vi "Load Virt Instrs.vi"(7 "Target Enqueuer":refnum<class "Message Enqueuer.lvclass">, 8 "error in":errorcluster, 10 "Virt Instrs":T1(array[cluster]), 11 "MSS in":refnum<class "Measure and Stimulus Subsystems.lvclass">) -> (0 "error out":errorcluster, 3 "MSS out":refnum<class "Measure and Stimulus Subsystems.lvclass">)   [LabVIEW 2023, in "HAL GOOP4.lvlib" / "Measure and Stimulus Subsystems.lvclass"]
uses:
  Measure and Stimulus Subsystems.lvclass
  <vilib>/ActorFramework/Message Enqueuer/Message Enqueuer.lvclass
  Measure and Stimulus Subsystems.lvclass/Measure and Stimulus Subsystems.ctl
  Virt Instr Host/Virt Instr Local.lvclass
  Virt Instr Base/Virt Instr Base.lvclass/Virt Instr Base.ctl
  <vilib>/Utility/miscctls.llb/LVMapReplaceAction.ctl
  Virt Instr Target/Virt Instr Target.lvclass
  MSS Target/IMSS Target Actor Messages/Init Virtual Instruments Msg/Init Virtual Instruments Msg.lvclass/Init Virtual Instruments Msg.ctl
  <vilib>/ActorFramework/Message Enqueuer/Message Enqueuer.lvclass/Message Enqueuer.ctl
  <vilib>/ActorFramework/Message Enqueuer/Enqueue.vi
  MSS Target/IMSS Target Actor Messages/Init Virtual Instruments Msg/Init Virtual Instruments Msg.lvclass
  <vilib>/Utility/LVClass/Get LV Class Name.vi
  <resource>/AFDebug/Generate Trace for Message.vi
  <vilib>/ActorFramework/Message Priority Queue/Priority Enqueue.vi
  Virt Instr Base/Virt Instr Base.lvclass
  D:/git/HAL/HAL GOOP4/Virt Instr Base/Virt Instr Base.lvclass
  D:/git/HAL/HAL GOOP4/Virt Instr Host/Virt Instr Local.lvclass
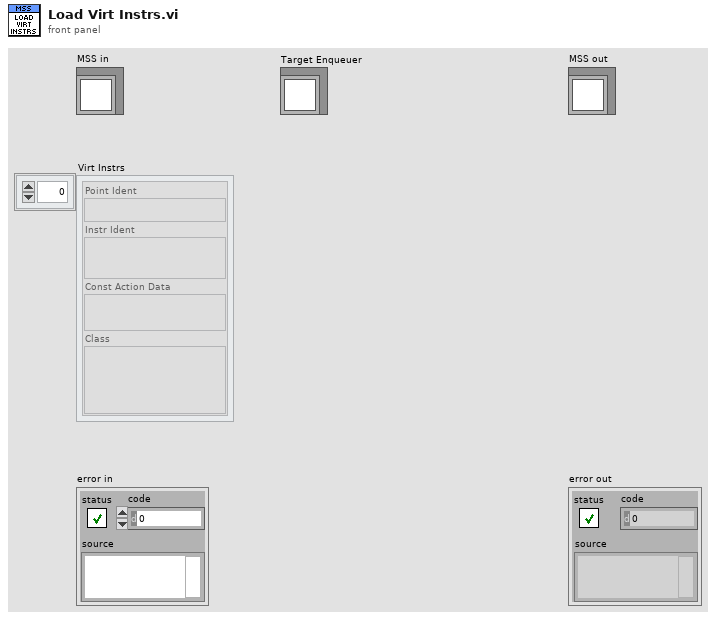
[diagram p1: front panel]
types:
  T1 = cluster{"Point Ident":string, "Instr Ident":string, "Const Action Data":string, "Class":string}[]
  T2 = typedef "LVMapReplaceAction.ctl" = enum32{"Modify Entry only if found", "Add or Modify Entry", "Delete Entry"}
  T3 = map{string, refnum<class "Virt Instr Local.lvclass">}
  T4 = map{string, cluster{"Instrument":refnum<class "Instrument.lvclass">, "Ref Count":u8}}
  T5 = cluster{"Instrument":refnum<class "Instrument.lvclass">, "Ref Count":u8}
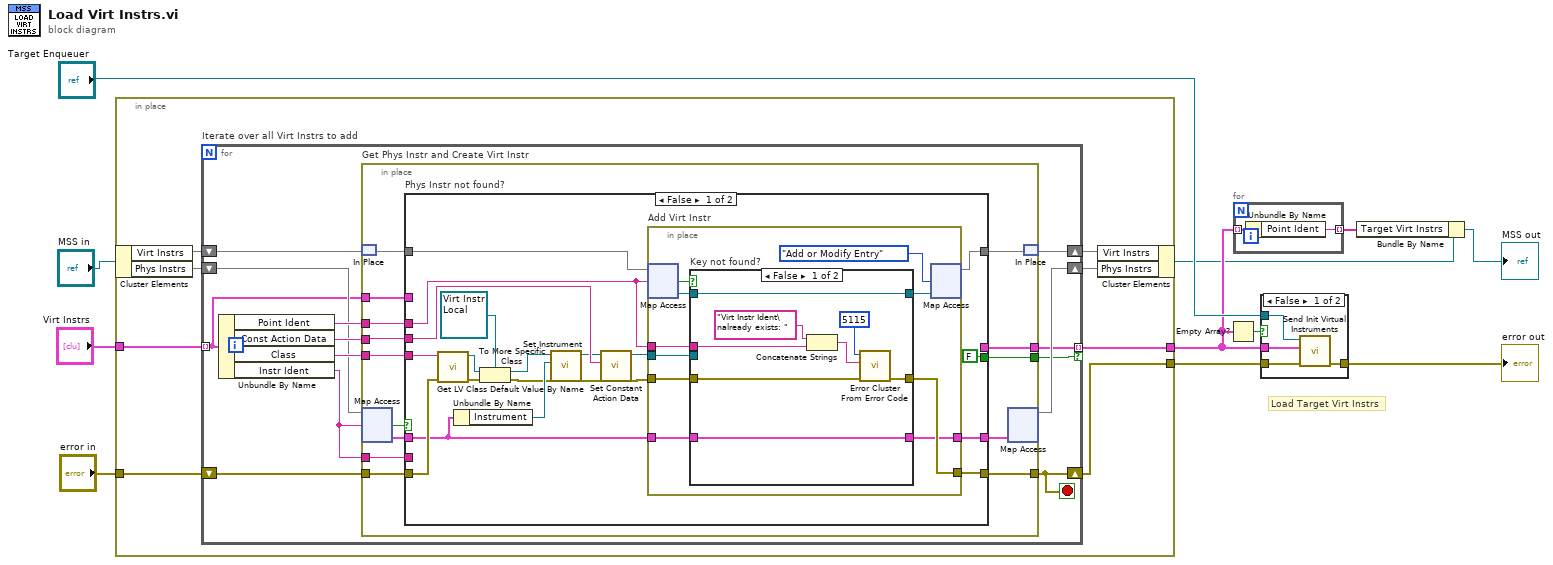
[diagram p0: block diagram]
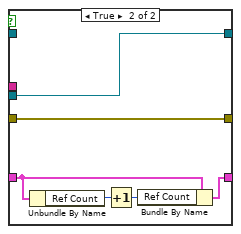
[diagram p2: hidden frame]
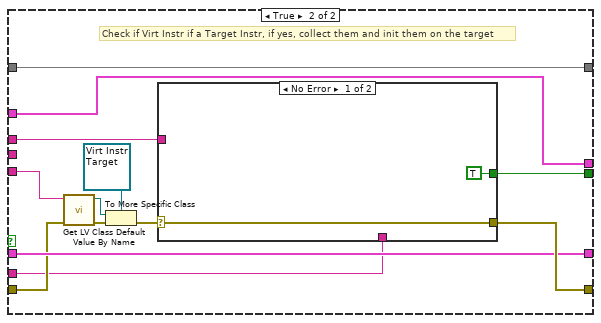
[diagram p3: hidden frame]
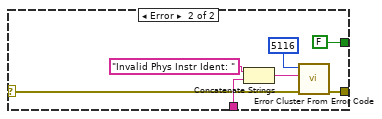
[diagram p4: hidden frame]
diagram:
  # "Load Target Virt Instrs"
  n1 = in-place {
    in-place-border: "error in" -> [w14]
    in-place-border: "Virt Instrs" -> [w19]
    in-place-border: [w13] -> w4
    in-place-border: [w12] -> w6
    n2 = in-place-cluster #1("MSS in") -> ("Virt Instrs"=w17:T3, "Phys Instrs"=w18:T4)
    n3 = for "Iterate over all Virt Instrs to add" {
      tunnel: w19 -> [w23] mode=indexing
      shift-right: [w29] -> w12
      shift-left: w14 -> [w31]
      shift-right: [w24] -> w15
      shift-left: w18 -> [w27]
      shift-right: [w25] -> w16
      shift-left: w17 -> [w26]
      tunnel: [w22] -> w13 mode=indexing if=w21
      stop <- w29 stop-if-true
      n4 = Unbundle By Name(w23) -> ("Point Ident"=w28:string, "Const Action Data"=w30:string, "Class"=w32:string, "Instr Ident"=w20:string)
      n5 = in-place "Get Phys Instr and Create Virt Instr" {
        in-place-border: w32 -> [w46]
        in-place-border: w31 -> [w45]
        in-place-border: w30 -> [w44]
        in-place-border: [w43] -> w29
        in-place-border: w28 -> [w42]
        in-place-border: w23 -> [w36]
        in-place-border: [w35] -> w22
        in-place-border: [w34] -> w21
        in-place-border: w20 -> [w33]
        n6 = in-place-match #2(w26) -> (w41:T3)
        n7 = in-place-map #3(w27, w20) -> (w39:T5, w37:bool)  [unwired: 1 in]
        n8 = case "Phys Instr not found?" shown="False" w37 {
          tunnel: w46 -> [w64 w97]
          tunnel: w45 -> [w63 w96]
          tunnel: w44 -> [w59 _]
          tunnel: [w56 w101] -> w43
          tunnel: w42 -> [w47 w91]
          tunnel: w41 -> [w53 w90]
          tunnel: [w58 w90] -> w40
          tunnel: w39 -> [w55 w100]
          tunnel: [w54 w100] -> w38
          tunnel: w36 -> [_ w93]
          tunnel: [_ w93] -> w35
          tunnel: [FALSE w92] -> w34
          tunnel: w33 -> [_ w89]
          frame False {
            n9 = call <vilib>:"Get LV Class Default Value By Name.vi"("error in (no error)"=w63, "class name"=w64) -> ("error out"=w62:errorcluster, "object"=w60:refnum<class>)  [unwired: 8 in]
            n10 = Unbundle By Name(w55) -> ("Instrument"=w51:refnum<class "Instrument.lvclass">)
            n11 = To More Specific Class(target class=refnum<class "Virt Instr Local.lvclass"> refnum ("Virt Instr Target"), reference=w60, error in=w62) -> (specific class reference=w50:refnum<class "Virt Instr Local.lvclass">, error out=w48:errorcluster)
            n12 = call "Set Instrument.vi"("HAL GOOP4.lvlib:Instrument"=w51, "Virt Instrument Base in"=w50) -> ("Virt Instrument Base out"=w52:refnum<class "Virt Instr Local.lvclass">)  [unwired: 9 in]
            n13 = call "Set Constant Action Data.vi"("Constant Action Data"=w59, "Virt Instr Base in"=w52) -> ("Virt Instr Base out"=w57:refnum<class "Virt Instr Local.lvclass">)  [unwired: 9 in]
            n14 = in-place "Add Virt Instr" {
              in-place-border: w57 -> [w72]
              in-place-border: w48 -> [w70]
              in-place-border: [w69] -> w56
              in-place-border: [w67] -> w54
              in-place-border: w55 -> [w66]
              in-place-border: w47 -> [w65]
              n15 = in-place-map #4(w53, w47) -> (w73:refnum<class "Virt Instr Local.lvclass">, w74:bool)  [unwired: 1 in]
              n16 = case "Key not found?" shown="False" w74 {
                tunnel: w73 -> [w81 _]
                tunnel: w72 -> [_ w83]
                tunnel: [w81 w83] -> w71
                tunnel: w70 -> [w82 w88]
                tunnel: [w79 w88] -> w69
                tunnel: w66 -> [w80 w85]
                tunnel: [w80 w84] -> w67
                tunnel: w65 -> [w75 _]
                frame False {
                  n17 = Concatenate Strings("Virt Instr Ident\nalready exists: " ("string"), w75) -> (w77:string)
                  n18 = call <vilib>:"Error Cluster From Error Code.vi"("error in (no error)"=w82, "error message (\"\")"=w77, "error code (0)"=5115) -> ("error out"=w79:errorcluster)  [unwired: 6 in]
                }
                frame True {
                  n19 = Unbundle By Name(w85) -> ("Ref Count"=w87:u8)
                  n20 = Increment(x=w87) -> (x+1=w86:u8)
                  n21 = Bundle By Name(cluster=w85, "Ref Count"=w86) -> (w84:T5)
                }
              }
              n22 = in-place-map #4(w71, LVMapReplaceAction."Add or Modify Entry" ("action")) -> (w58:T3)  [unwired: 2 out]
            }
          }
          frame True {
            # "Check if Virt Instr if a Target Instr, if yes, collect them and init them on the target"
            n23 = call <vilib>:"Get LV Class Default Value By Name.vi"("error in (no error)"=w96, "class name"=w97) -> ("error out"=w95:errorcluster, "object"=w99:refnum<class>)  [unwired: 8 in]
            n24 = To More Specific Class(target class=refnum<class "Virt Instr Target.lvclass"> refnum ("Virt Instr Target"), reference=w99, error in=w95) -> (error out=w94:errorcluster)  [unwired: 1 out]
            n25 = case shown="No Error" w94 {
              selector: w94 -> [w102 w104]
              tunnel: [w102 w110] -> w101
              tunnel: [TRUE FALSE] -> w92
              tunnel: w91 -> [_ _]
              tunnel: w89 -> [_ w106]
              frame No Error {
              }
              frame Error {
                n26 = Concatenate Strings("Invalid Phys Instr Ident: " ("string"), w106) -> (w105:string)
                n27 = call <vilib>:"Error Cluster From Error Code.vi"("error in (no error)"=w104, "error message (\"\")"=w105, "error code (0)"=5116) -> ("error out"=w110:errorcluster)  [unwired: 6 in]
              }
            }
          }
        }
        n28 = in-place-map #3(w38) -> (w24:T4)  [unwired: 1 in, 2 out]
        n29 = in-place-match #2(w40) -> (w25:T3)
      }
    }
    n30 = in-place-cluster #1("Virt Instrs"=w16, "Phys Instrs"=w15) -> (w3:refnum<class "Measure and Stimulus Subsystems.lvclass">)
  }
  n31 = Empty Array?(array=w4) -> (empty?=w8:bool)
  n32 = for {
    tunnel: [w112] -> w1 mode=indexing
    tunnel: w4 -> [w111] mode=indexing
    n33 = Unbundle By Name(w111) -> ("Point Ident"=w112:string)
  }
  n34 = case shown="False" w8 {
    tunnel: "Target Enqueuer" -> [w116 _]
    tunnel: w6 -> [w115 w117]
    tunnel: [w114 w117] -> w5
    tunnel: w4 -> [w113 _]
    frame False {
      n35 = call "Send Init Virtual Instruments.vi"("error in (no error)"=w115, "Virt Instrs"=w113, "Message Enqueuer"=w116) -> ("error out"=w114:errorcluster)  [unwired: 7 in, 1 out]
    }
    frame True {
    }
  }
  "error out" <- w5
  n36 = Bundle By Name(cluster=w3, "Target Virt Instrs"=w1) -> (→"MSS out":refnum<class "Measure and Stimulus Subsystems.lvclass">)
